vi "Test EEPROM.vi"() -> ()   [LabVIEW 2015]
doc: "Created IvanLis by LabVIEW Portal\nProfile: http://labviewportal.org/memberlist.php?mode=viewprofile&u=987\neMail: IvanLisanov@gMail.com\nTelegram: https://t.me/IvanLis"
uses:
  RTL-SDR Class/RTL-SDR.lvclass
panel:
  out "Length":u16
  out "Data Out":u8[](array[numeric])
  in  "Length Out":u16
  in  "Offset Out":u8
  in  "Read":bool
  out "Length In":u16
  in  "Offset In":u8
  in  "Data In":u8[](array[numeric])
  in  "Write":bool
  in  "Device Index":u32=1
  in  "Open":bool
  in  "stop":bool
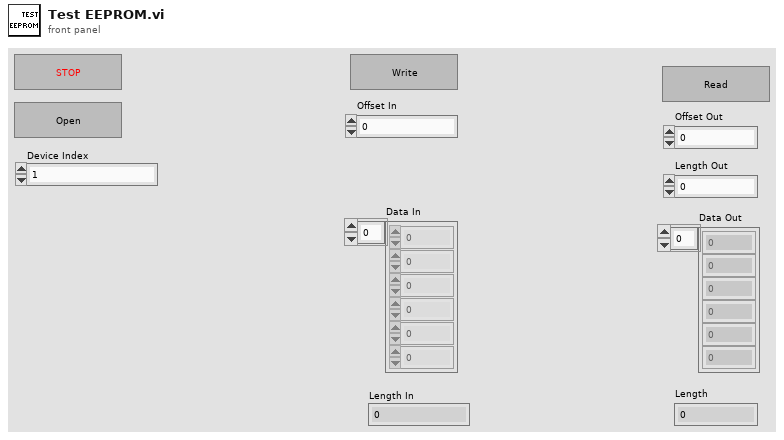
[diagram p1: front panel]
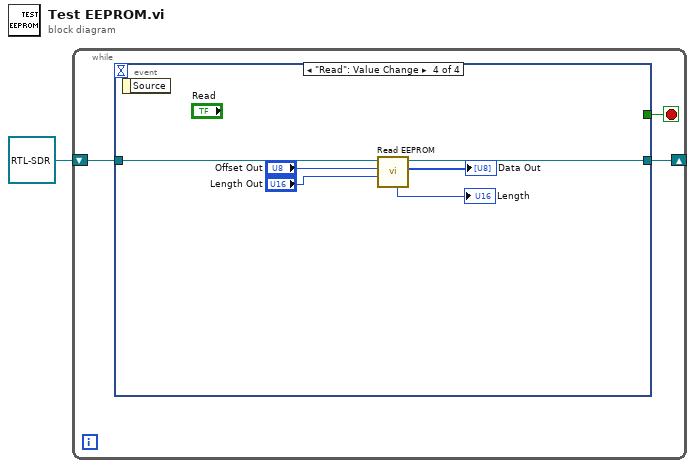
[diagram p0: block diagram]
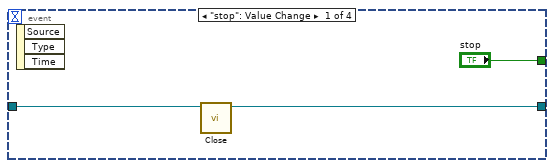
[diagram p2: hidden frame]
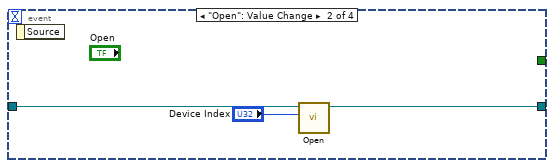
[diagram p3: hidden frame]
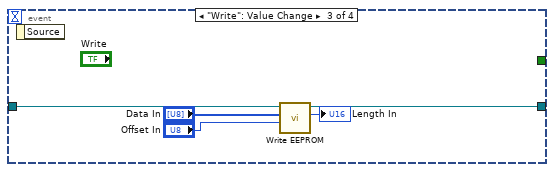
[diagram p4: hidden frame]
diagram:
  n1 = while {
    shift-right: [w2] -> _
    shift-left: refnum<class "RTL-SDR.lvclass"> refnum ("RTL-SDR in") -> [w3]
    stop <- w4 stop-if-true
    n2 = event shown="[3] \"Read\": Value Change" {
      selector: _ -> [_ _ _ _]
      dyn-events: _ -> [_ _ _ _]
      timeout: _ -> [_ _ _ _]
      tunnel: ["stop" _ _ _] -> w4
      tunnel: w3 -> [w6 w10 w15 w21]
      tunnel: [w5 w9 w14 w20] -> w2
      event "stop": Value Change {
        n3 = event-data() -> ()  [unwired: 1 in, 3 out]
        n4 = call "Close.vi"("RTL-SDR in"=w6) -> ("RTL-SDR out"=w5:refnum<class "RTL-SDR.lvclass">)  [unwired: 8 in, 2 out]
      }
      event "Open": Value Change {
        n5 = event-data() -> ()  [unwired: 1 in, 1 out]
        n6 = call "Open.vi"("Device Index"="Device Index", "RTL-SDR in"=w10) -> ("RTL-SDR out"=w9:refnum<class "RTL-SDR.lvclass">)  [unwired: 7 in, 2 out]
      }
      event "Write": Value Change {
        n7 = event-data() -> ()  [unwired: 1 in, 1 out]
        n8 = call "Write EEPROM.vi"("Offset"="Offset In", "Data"="Data In", "RTL-SDR in"=w15) -> ("Length"=→"Length In":u16, "RTL-SDR out"=w14:refnum<class "RTL-SDR.lvclass">)  [unwired: 5 in, 2 out]
      }
      event "Read": Value Change {
        n9 = event-data() -> ()  [unwired: 1 in, 1 out]
        n10 = call "Read EEPROM.vi"("Length In"="Length Out", "Offset In"="Offset Out", "RTL-SDR in"=w21) -> ("Data"=→"Data Out":u8[], "RTL-SDR out"=w20:refnum<class "RTL-SDR.lvclass">, "Length"=→"Length":u16)  [unwired: 4 in, 2 out]
      }
    }
  }
